vi "Stop Core.vi"(10 "final error code":i32, 11 "cRIO Vacuum in":refnum<class "cRIO Vacuum.lvclass">) -> (3 "cRIO Vacuum out":refnum<class "cRIO Vacuum.lvclass">)   [LabVIEW 2015, in "cRIO-Carbondioxide.lvlib" / "CO2-Actor.lvlib" / "cRIO Vacuum.lvclass"]
doc: "(<B>Filename</B>: Actor Framework.lvlib:Actor.lvclass:Stop Core.vi)\n\nDefines what the actor does before it stops. Use the <B>final error code</B> input to determine whether the actor shut down in response to an error.\n\nBy default, this method does nothing. A descendant class may override it to define behavior, such as shutting down any processes the actor initiated in its override of the Actor Core method."
uses:
  cRIO Vacuum.lvclass
  cRIO Vacuum.lvclass/cRIO Vacuum.ctl
  <vilib>/ActorFramework/Time-Delayed Send Message/Time-Delay Override Options.ctl
  CO2 Actor/CO2 Actor.lvclass
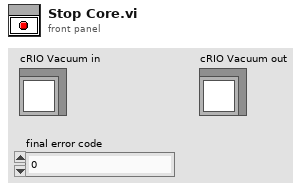
[diagram p1: front panel]
types:
  T1 = typedef "Time-Delay Override Options.ctl" = enum16{"Send next copy now", "Skip next scheduled copy", "Send next copy now and stop all further copies", "Stop all further copies"}
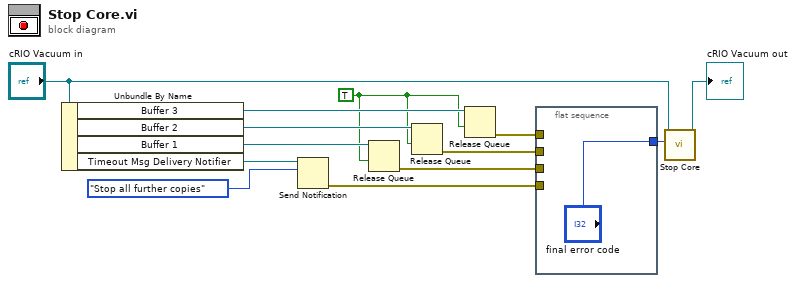
[diagram p0: block diagram]
diagram:
  w2 = TRUE ("force destroy? (F)")
  n1 = Unbundle By Name("cRIO Vacuum in") -> ("Buffer 3"=w3:refnum<queue>, "Buffer 2"=w8:refnum<queue>, "Buffer 1"=w5:refnum<queue>, "Timeout Msg Delivery Notifier"=w11:refnum<notifier>)
  n2 = Send Notification(notification=Time-Delay_Override_Options."Stop all further copies", notifier=w11) -> (error out=w6:errorcluster)  [unwired: 1 in, 1 out]
  n3 = Release Queue(queue=w5, force destroy? (F)=w2) -> (error out=w4:errorcluster)  [unwired: 1 in, 2 out]
  n4 = Release Queue(queue=w8, force destroy? (F)=w2) -> (error out=w7:errorcluster)  [unwired: 1 in, 2 out]
  n5 = Release Queue(queue=w3, force destroy? (F)=w2) -> (error out=w1:errorcluster)  [unwired: 1 in, 2 out]
  n6 = flat-sequence {
    tunnel: ["final error code"] -> w9
    tunnel: w7 -> [_]
    tunnel: w6 -> [_]
    tunnel: w4 -> [_]
    tunnel: w1 -> [_]
    frame #0 {
    }
  }
  n7 = call-parent "Stop Core.vi"("final error code"=w9, "CO2 Actor in"="cRIO Vacuum in") -> ("CO2 Actor out"=→"cRIO Vacuum out":refnum<class "cRIO Vacuum.lvclass">)  [unwired: 9 in]
